vi "sm u64 read array and increment.vi"(9 "Identifier":string="default", 10 "array size":u64, 11 "Shared memory cluster":T1) -> (2 "value out":u64[](array[numeric]), 3 "Shared memory cluster output":T1)   [LabVIEW 2020, in "linuxSharedMemory.lvlib"]
uses:
  linuxSharedMemory.lvlib
  controls/sm_cluster.ctl
  <vilib>/NI/NI Linux RT IPC/Shared Memory/Pointer Operations/Read 1D Array U64.vi
  <vilib>/NI/NI Linux RT IPC/Shared Memory/Pointer Operations/In Place Read 1D Array U64.vi
  <vilib>/NI/NI Linux RT IPC/Shared Memory/Linux RT IPC.Shared Memory.lvlib
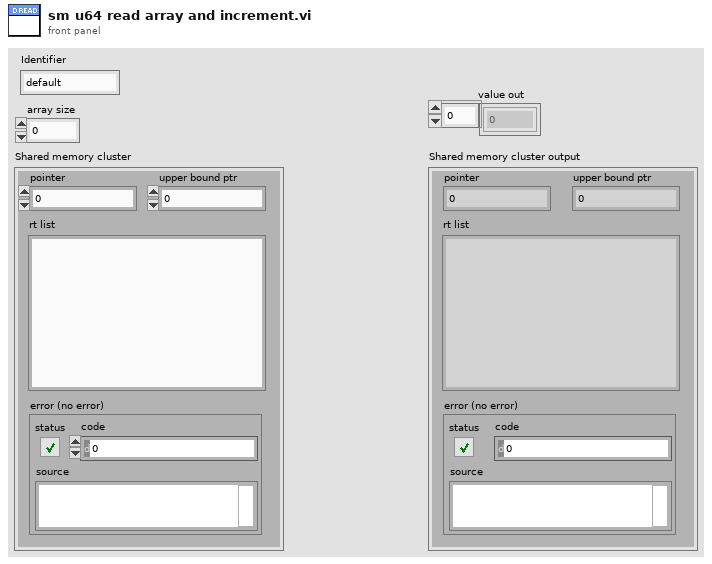
[diagram p1: front panel]
types:
  T1 = typedef "linuxSharedMemory.lvlib/sm_cluster.ctl" = cluster{"rt list":string, "error (no error)":errorcluster, "pointer":u64, "upper bound ptr":u64}
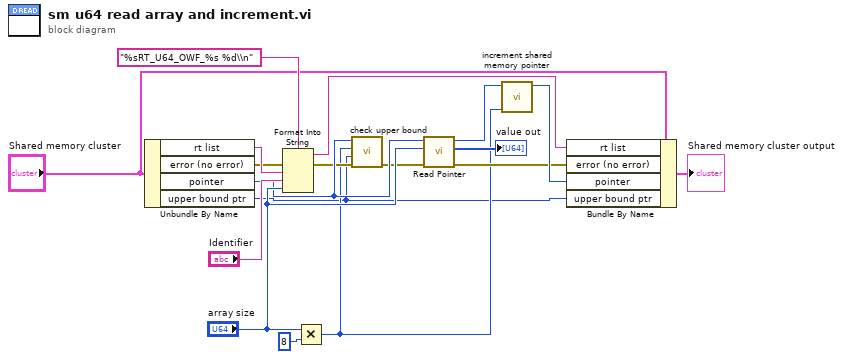
[diagram p0: block diagram]
diagram:
  n1 = Unbundle By Name("Shared memory cluster") -> ("rt list"=w14:string, "error (no error)"=w9:errorcluster, "pointer"=w7:u64, "upper bound ptr"=w1:u64)
  n2 = Format Into String(format string="%sRT_U64_OWF_%s %d\\n", error in=w9, w14, "Identifier", "array size") -> (resulting string=w11:string, error out=w6:errorcluster)  [unwired: 1 in]
  n3 = Multiply(x="array size", y=8) -> (x*y=w2:u64)
  n4 = call "check upper bound.vi"("error in (no error)"=w6, "ptr upper bound (inclusive)"=w1, "size"=w2, "ptr in"=w7) -> ("error out"=w5:errorcluster)  [unwired: 7 in]
  n5 = call-poly <vilib>:"Read Pointer.vi"("error in (no error)"=w5, "number of elements"="array size", "pointer in"=w7) -> ("error out"=w12:errorcluster, "value"=→"value out":u64[], "pointer out"=w18:u64)  [unwired: 5 in, 1 out]
  n6 = call "increment shared memory pointer.vi"("Increment value"=w2, "Shared Memory PTR in"=w18) -> ("Shared Memory PTR out"=w13:u64)  [unwired: 9 in]
  n7 = Bundle By Name(cluster="Shared memory cluster", "rt list"=w11, "error (no error)"=w12, "pointer"=w13, "upper bound ptr"=w1) -> (→"Shared memory cluster output":T1)
